vi "Get Process by Index.vi"(8 "error in (no error)":errorcluster, 10 "Select Module":i32, 11 "Application in":refnum<class "Application.lvclass">) -> (0 "error out":errorcluster, 2 "Processes":refnum<class "Process.lvclass">[](array[class]), 3 "Application out":refnum<class "Application.lvclass">)   [LabVIEW 2020]
uses:
  <vilib>/Asteme/Triarc Framework/Process/Process.lvclass
  <vilib>/Asteme/Triarc Framework/Application/Application.lvclass
  C:/Program Files (x86)/National Instruments/LabVIEW 2020/vi.lib/Asteme/Triarc Framework/Process/Process.lvclass
  <vilib>/Asteme/Triarc Framework/Process/Process.lvclass/Process.ctl
  <vilib>/Asteme/Triarc Framework/Application/Application.lvclass/Application.ctl
  <vilib>/Asteme/Triarc Framework/Process/Public/Lifecycle/Get Lifecycle State.vi
  <vilib>/Asteme/Triarc Framework/Process/Protected/Messaging/Request Message.vi
  <vilib>/Utility/error.llb/Clear Errors.vi
  <vilib>/Asteme/Triarc Framework/Process/Private/SubVIs/Enqueue Request Message.vi
  <vilib>/Utility/error.llb/Error Cluster From Error Code.vi
  <vilib>/Asteme/Triarc Framework/Process/Private/SubVIs/Wait for Response Message.vi
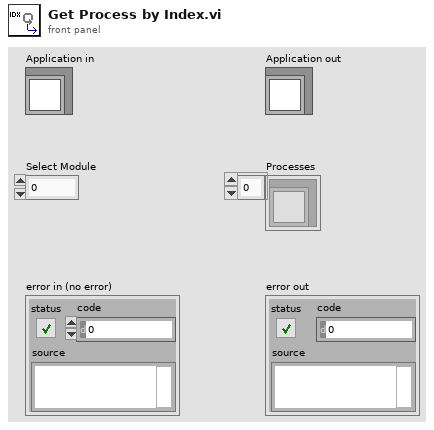
[diagram p1: front panel]
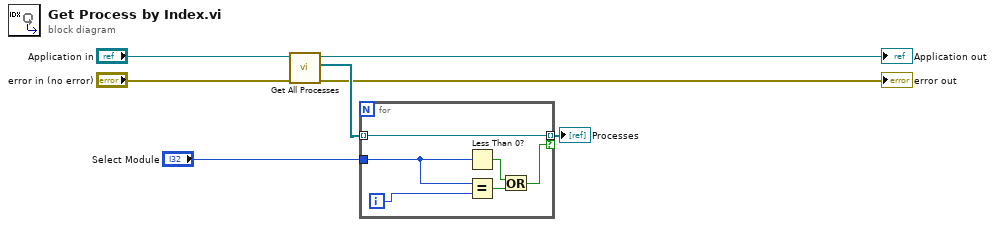
[diagram p0: block diagram]
diagram:
  n1 = call <vilib>:"Get All Processes.vi"("error in (no error)"="error in (no error)", "Application In"="Application in") -> ("error out"=→"error out":errorcluster, "App Processes"=w5:refnum<class "Process.lvclass">[], "Application Out"=→"Application out":refnum<class "Application.lvclass">)  [unwired: 7 in]
  n2 = for {
    tunnel: w5 -> [w13] mode=indexing
    tunnel: [w13] -> w6 mode=indexing if=w8
    tunnel: "Select Module" -> [w9]
    i -> [w12]
    n3 = Less Than 0?(x=w9) -> (x < 0?=w10:bool)
    n4 = Equal?(x=w9, y=w12) -> (x = y?=w11:bool)
    n5 = Or(x=w10, y=w11) -> (x .or. y?=w8:bool)
  }
  "Processes" <- w6
